vi "Video Upload.vi"(0 "Sift Client in":refnum<class "Sift Client.lvclass">, 1 "Filepath":string, 2 "Entity ID":string, 3 "Entity Type":T1, 4 "Description":string, 5 "error in (no error)":errorcluster, 6 "Timestamp":timestamp, 7 "Width":i32, 8 "Duration (s)":dbl, 9 "Height":i32, 11 "Timeout (ms) (60000)":i32=60000) -> (14 "Sift Client out":refnum<class "Sift Client.lvclass">, 19 "error out":errorcluster)   [LabVIEW 2024, in "Sift Client.lvlib" / "Sift Client.lvclass"]
doc: "Uploads a file pointed to by Filepath and attaches it to the provided Entity ID. Optionally include the video width, height, duration, and timestamp for optimal viewing experience in the Sift application.\n\nBy default will wait 60s for the upload to take place. Increase this time by setting the Timeout if needed."
uses:
  Sift Client.lvclass
  Private/Typedefs/Messages/File Attachment Upload Request.ctl
  Types/Entity Type.ctl
  Private/Typedefs/Messages/Video Metadata.ctl
  Private/Typedefs/Messages/Image Metadata.ctl
  Private/Typedefs/Messages/Metadata Type.ctl
  Private/Typedefs/Messages/JSON Request.ctl
  Sift Client.lvclass/Sift Client.ctl
  Sift Client.lvlib
  <vilib>/addons/_JKI.lib/Serialization/JSON/JKI JSON Serialization.lvlib
panel:
  in  "video_metadata":T2
  in  "JSON Request":T3
  in  "File Attachment Upload Request":T4
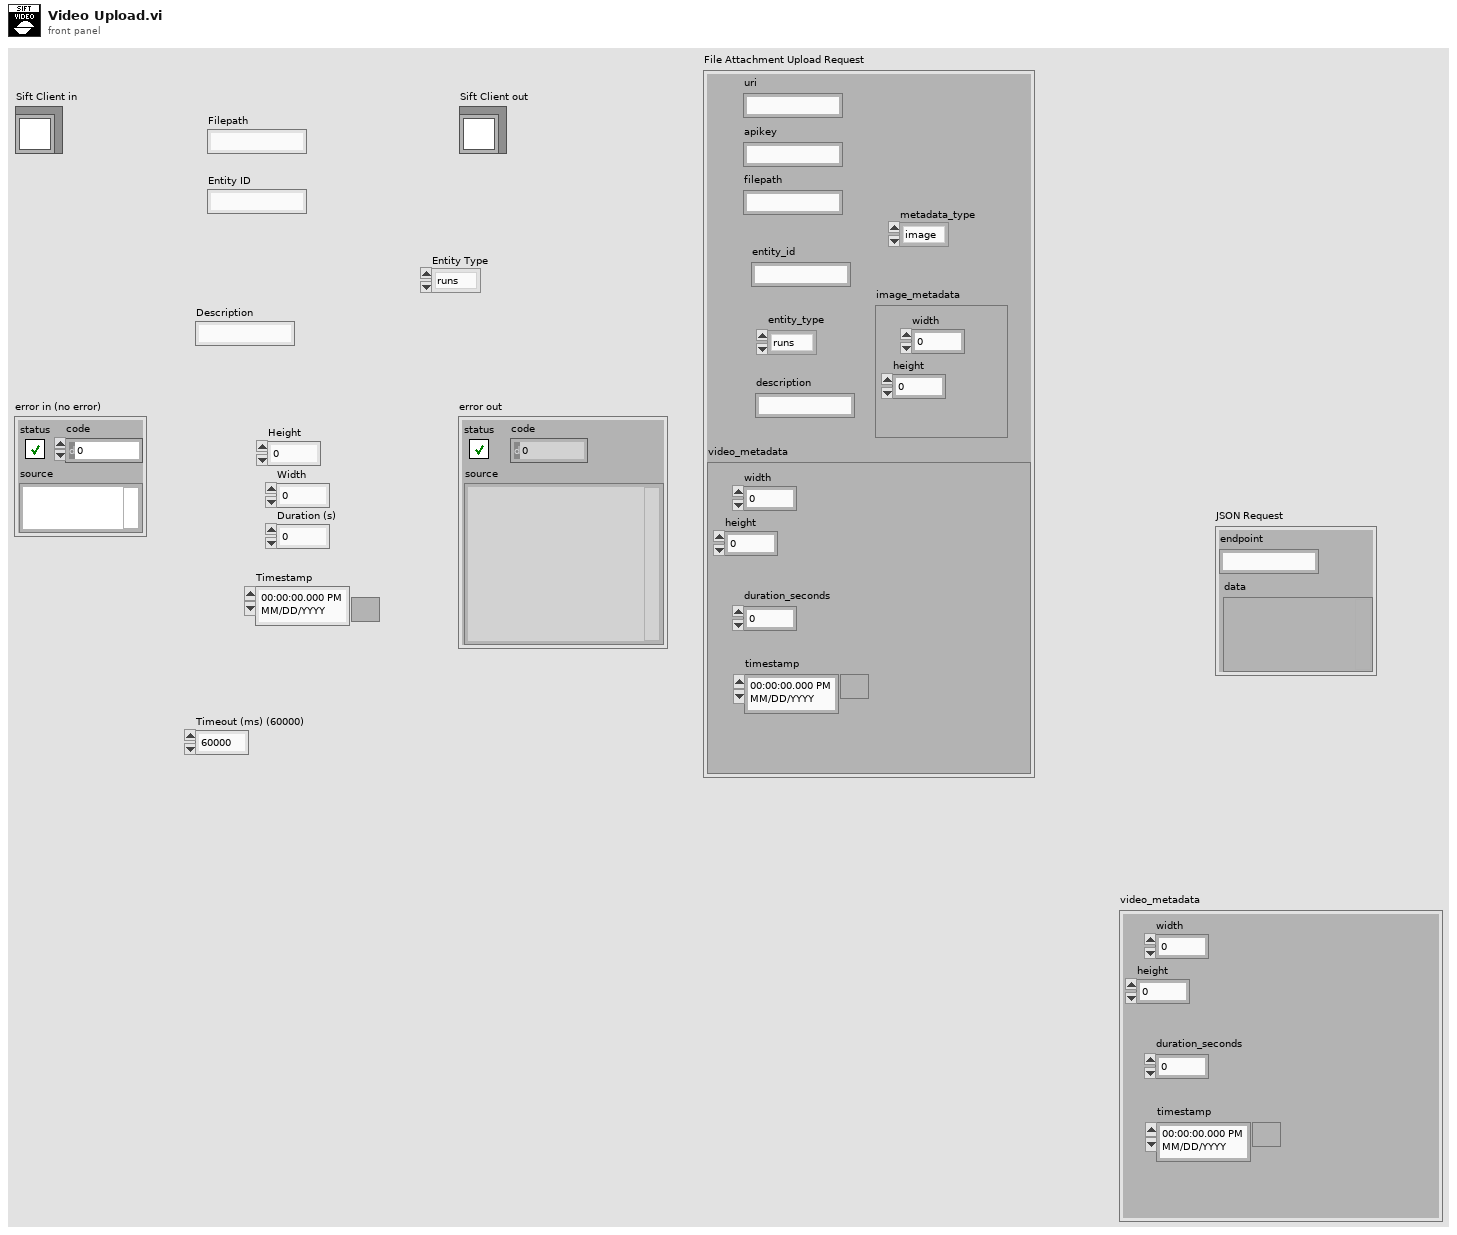
[diagram p1: front panel]
types:
  T1 = typedef "Sift Client.lvlib/Entity Type.ctl" = enum16{"runs", "annotations", "annotation_logs"}
  T2 = typedef "Sift Client.lvlib/Video Metadata.ctl" = cluster{"duration_seconds":dbl, "timestamp":timestamp, "height":i32, "width":i32}
  T3 = typedef "Sift Client.lvlib/JSON Request.ctl" = cluster{"endpoint":string, "data":variant}
  T4 = typedef "Sift Client.lvlib/File Attachment Upload Request.ctl" = cluster{"uri":string, "apikey":string, "filepath":string, "entity_id":string, "description":string, "entity_type":T1, "video_metadata":T2, "image_metadata":T5, "metadata_type":T6}
  T5 = typedef "Sift Client.lvlib/Image Metadata.ctl" = cluster{"height":i32, "width":i32}
  T6 = typedef "Sift Client.lvlib/Metadata Type.ctl" = enum16{"image", "video"}
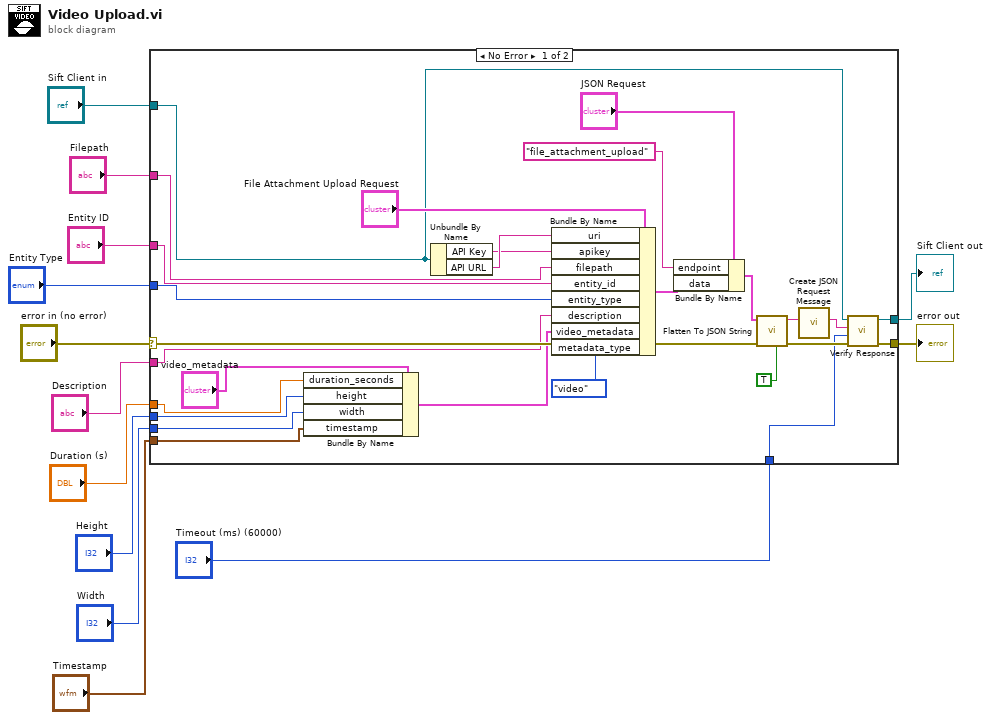
[diagram p0: block diagram]
diagram:
  n1 = case shown="No Error" "error in (no error)" {
    selector: "error in (no error)" -> [w32 w42]
    tunnel: [w31 w42] -> w12
    tunnel: [w30 w41] -> w10
    tunnel: "Sift Client in" -> [w29 w41]
    tunnel: "Entity Type" -> [w26 _]
    tunnel: "Entity ID" -> [w25 _]
    tunnel: "Filepath" -> [w24 _]
    tunnel: "Description" -> [w23 _]
    tunnel: "Height" -> [w22 _]
    tunnel: "Width" -> [w21 _]
    tunnel: "Duration (s)" -> [w20 _]
    tunnel: "Timestamp" -> [w19 _]
    tunnel: "Timeout (ms) (60000)" -> [w14 _]
    frame No Error {
      n2 = Bundle By Name(cluster="video_metadata", "duration_seconds"=w20, "height"=w22, "width"=w21, "timestamp"=w19) -> (w18:T2)
      n3 = Unbundle By Name(w29) -> ("API Key"=w27:string, "API URL"=w28:string)
      n4 = Bundle By Name(cluster="File Attachment Upload Request", "uri"=w28, "apikey"=w27, "filepath"=w24, "entity_id"=w25, "entity_type"=w26, "description"=w23, "video_metadata"=w18, "metadata_type"=Metadata_Type."video") -> (w38:T4)
      n5 = Bundle By Name(cluster="JSON Request", "endpoint"="file_attachment_upload", "data"=w38) -> (w33:T3)
      n6 = call <vilib>:"Flatten To JSON String.vi"("Enums As String (F)"=TRUE, "error in"=w32, "Variant"=w33) -> ("error out"=w34:errorcluster, "JSON String"=w36:string)  [unwired: 7 in]
      n7 = call "Create JSON Request Message.vi"("Data"=w36) -> ("Message"=w35:string)  [unwired: 10 in]
      n8 = call-dynamic "Verify Response.vi"("error in (no error)"=w34, "timeout ms (25000)"=w14, "Message"=w35, "Sift Client in"=w29) -> ("error out"=w31:errorcluster, "Sift Client out"=w30:refnum<class "Sift Client.lvclass">)  [unwired: 5 in, 1 out]
    }
    frame Error {
    }
  }
  "error out" <- w12
  "Sift Client out" <- w10
